vi "DriveSetRobotPosition.vi"(2 "Parameter String":string, 3 "Reinit":bool) -> (0 "Error Out":errorcluster, 1 "Increment":bool)   [LabVIEW 2020]
doc: "This VI sets the robot position. This can be used to zero out accumulated position error based on a fiducial.\n\nParameters:\n1. X location --> (in) [15,614.25]\n2. Y location --> (in) [15,308.25]"
uses:
  SafeParser_Float.vi
  sensordata.vi
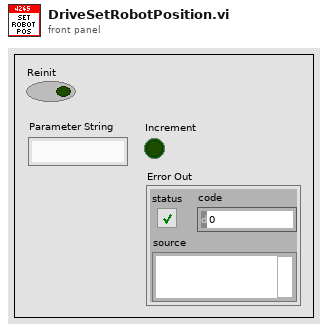
[diagram p1: front panel]
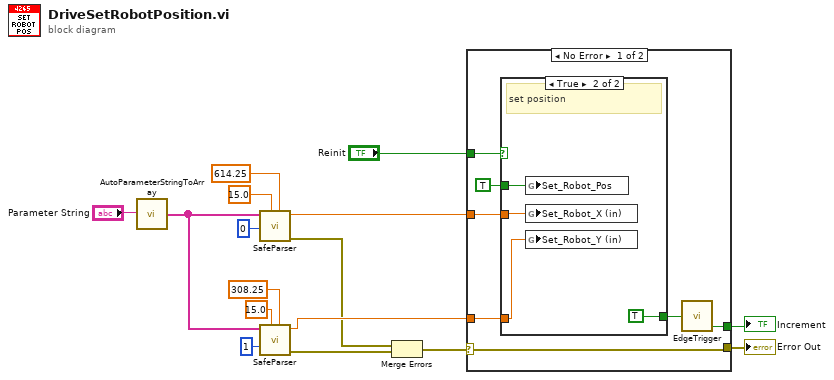
[diagram p0: block diagram]
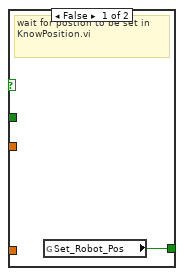
[diagram p2: hidden frame]
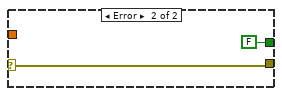
[diagram p3: hidden frame]
diagram:
  n1 = call "AutoParameterStringToArray.vi"("Parameter String"="Parameter String") -> ("Parsed Parameters"=w9:string[])
  n2 = call-poly "SafeParser.vi"("Maximum"=614.25, "Minimum"=15.0, "Array Index"=0 ("Parameter Index"), "String Array"=w9) -> ("Error Out"=w3:errorcluster, "Typecast  Value"=w5:dbl)  [unwired: 6 in]
  n3 = call-poly "SafeParser.vi"("Maximum"=308.25, "Minimum"=15.0, "Array Index"=1 ("Parameter Index"), "String Array"=w9) -> ("Error Out"=w6:errorcluster, "Typecast  Value"=w4:dbl)  [unwired: 6 in]
  n4 = Merge Errors(w3, w6) -> (w7:errorcluster)
  n5 = case shown="No Error" w7 {
    selector: w7 -> [w18 w30]
    tunnel: "Reinit" -> [w23 _]
    tunnel: w5 -> [w22 _]
    tunnel: [w19 FALSE ("Falling Edge Trigger")] -> w15
    tunnel: [w18 w30] -> w14
    tunnel: w4 -> [w17 _]
    frame No Error {
      n6 = case shown="True" w23 {
        tunnel: w22 -> [_ w28]
        tunnel: [w24 TRUE ("Falling Edge Trigger")] -> w20
        tunnel: TRUE -> [_ w26]
        tunnel: w17 -> [_ w25]
        frame False {
          # "wait for postion to be set in KnowPosition.vi"
          n7 = global read "sensordata.vi" "Set_Robot_Pos"() -> (w24:bool)
        }
        frame True {
          # "set position"
          n8 = global write "sensordata.vi" "Set_Robot_Pos"(w26) -> ()
          n9 = global write "sensordata.vi" "Set_Robot_X (in)"(w28) -> ()
          n10 = global write "sensordata.vi" "Set_Robot_Y (in)"(w25) -> ()
        }
      }
      n11 = call "EdgeTrigger.vi"("Input Signal"=w20) -> ("Falling Edge Trigger"=w19:bool)  [unwired: 2 out]
    }
    frame Error {
    }
  }
  "Increment" <- w15
  "Error Out" <- w14
